vi "_System Polling.vi"   [LabVIEW 2015]
uses:
  <vilib>/rvi/Emulation/niFpgaGetClockAttributes.vi
  <vilib>/rvi/Emulation/niFpgaSctlEmulationGetInTimedLoop.vi
  <vilib>/rvi/Emulation/niFpgaEmulationReportErrorSimple.vi
  <vilib>/rvi/Emulation/niFpgaCriticalErrorInLSC.vi
  <vilib>/rvi/DataTransferAndStorage/Container/XNode/niFpgaContainer.xnode
  <vilib>/rvi/Memory/Memory_Emulation/nirvimemoryEmulation.vi
  <vilib>/rvi/Memory/Memory_Emulation/nirvimemoryFastEmulation.vi
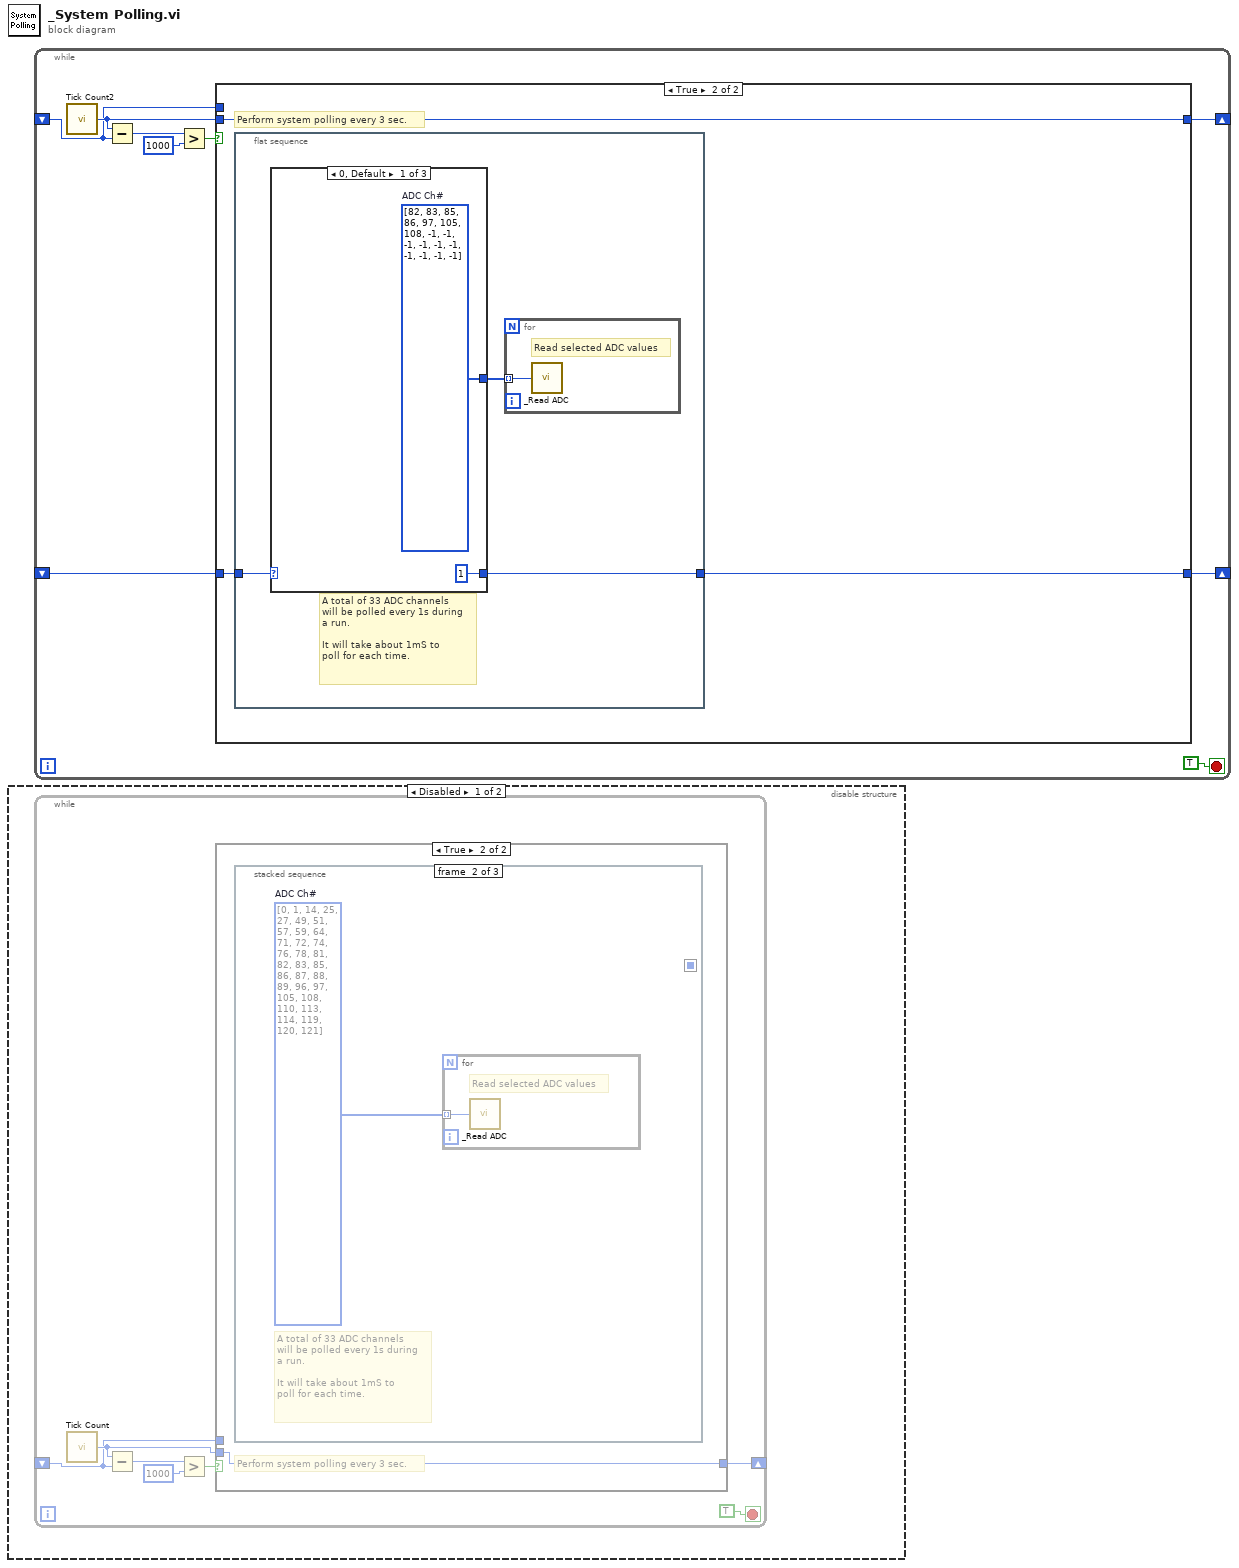
[diagram p0: block diagram]
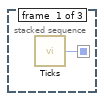
[diagram p3: hidden frame]
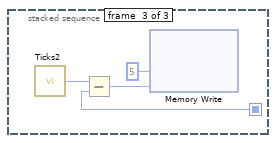
[diagram p4: hidden frame]
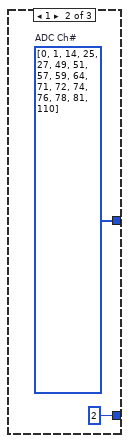
[diagram p7: hidden frame]
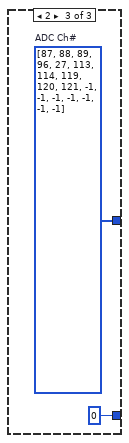
[diagram p8: hidden frame]
diagram:
  n1 = disable-structure shown="Disabled" {
    frame Disabled {
      n2 = while {
        shift-right: [w1] -> _
        shift-left: _ -> [w2]
        stop <- TRUE stop-if-true
        n3 = call "Tick Count"() -> ("Tick Count(mSec)"=w3:u32)
        n4 = Subtract(x=w3, y=w2) -> (x-y=w6:u32)
        n5 = Greater?(x=w6, y=u32 1000) -> (0:w4:bool)
        n6 = case shown="True" w4 {
          tunnel: w3 -> [_ w9]
          tunnel: w2 -> [w8 _]
          tunnel: [w8 w9] -> w1
          frame False {
          }
          frame True {
            # "Perform system polling every 3 sec."
            n7 = stacked-sequence {
              seq-local: [w10 _ _] -> [_ _ w13]
              frame #0 {
                n8 = call "Ticks"() -> ("Tick Count(Ticks)"=w10:u16)
              }
              frame #1 {
                w11 = u8[] [0, 1, 14, 25, 27, 49, 51, 57, 59, 64, 71, 72, 74, 76, 78, 81, 82, 83, 85, 86, 87, 88, 89, 96, 97, 105, 108, 110, 113, 114, 119, 120, 121]  # ADC Ch#
                # "A total of 33 ADC channels\nwill be polled every 1s during\na run.\n\nIt will take about 1mS to\npoll for each time."
                n9 = for {
                  tunnel: w11 -> [w12] mode=indexing
                  # "Read selected ADC values"
                  n10 = call "_Read ADC.vi"("Channel #"=w12) -> ()  [unwired: 1 out]
                }
              }
              frame #2 {
                n11 = call "Ticks2"() -> ("Tick Count(Ticks)"=w14:u16)
                n12 = Subtract(x=w14, y=w13) -> (x-y=w16:u16)
                n13 = xnode ("Memory Write")("Address"=u8 5, "Data"=w16) -> ()  [unwired: 1 in, 1 out]
              }
            }
          }
        }
      }
    }
    frame Enabled {
    }
  }
  n14 = while {
    shift-right: [w19] -> _
    shift-left: _ -> [w20]
    shift-right: [w17] -> _
    shift-left: _ -> [w18]
    stop <- TRUE stop-if-true
    n15 = call "Tick Count2"() -> ("Tick Count(mSec)"=w21:u32)
    n16 = Subtract(x=w21, y=w20) -> (x-y=w24:u32)
    n17 = Greater?(x=w24, y=u32 1000) -> (0:w22:bool)
    n18 = case shown="True" w22 {
      tunnel: w21 -> [_ w30]
      tunnel: w20 -> [w27 _]
      tunnel: [w27 w30] -> w19
      tunnel: w18 -> [w26 w29]
      tunnel: [w26 w28] -> w17
      frame False {
      }
      frame True {
        # "Perform system polling every 3 sec."
        n19 = flat-sequence {
          tunnel: [w31] -> w28
          tunnel: w29 -> [w32]
          frame #0 {
            # "A total of 33 ADC channels\nwill be polled every 1s during\na run.\n\nIt will take about 1mS to\npoll for each time."
            n20 = case shown="0, Default" w32 {
              tunnel: [w35 w37 w39] -> w33
              tunnel: [u32 1 ("y") u32 2 ("y") u32 0 ("y")] -> w31
              frame 0, Default {
                w35 = i8[] [82, 83, 85, 86, 97, 105, 108, -1, -1, -1, -1, -1, -1, -1, -1, -1, -1]  # ADC Ch#
              }
              frame 1 {
                w37 = i8[] [0, 1, 14, 25, 27, 49, 51, 57, 59, 64, 71, 72, 74, 76, 78, 81, 110]  # ADC Ch#
              }
              frame 2 {
                w39 = i8[] [87, 88, 89, 96, 27, 113, 114, 119, 120, 121, -1, -1, -1, -1, -1, -1, -1]  # ADC Ch#
              }
            }
            n21 = for {
              tunnel: w33 -> [w40] mode=indexing
              # "Read selected ADC values"
              n22 = call "_Read ADC.vi"("Channel #"=w40) -> ()  [unwired: 1 out]
            }
          }
        }
      }
    }
  }
